vi "ActualizarFrecuencia.vi"(8 "error in (no error)":errorcluster, 11 "Prueba031 in":refnum<class "Prueba03.lvclass">) -> (0 "error out":errorcluster, 1 "newFrec":string, 3 "Prueba031 out":refnum<class "Prueba03.lvclass">)   [LabVIEW 2019, in "Prueba03.lvclass"]
uses:
  Prueba03.lvclass
  Prueba03.lvclass/Prueba03.ctl
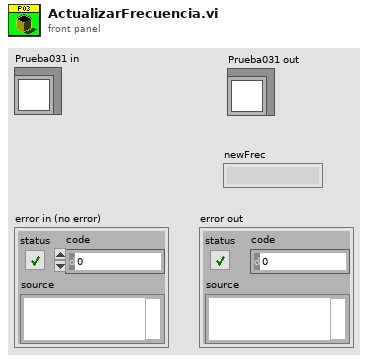
[diagram p1: front panel]
types:
  T1 = cluster{"ControlName":string, "ControlReference":refnum<vi>}[]
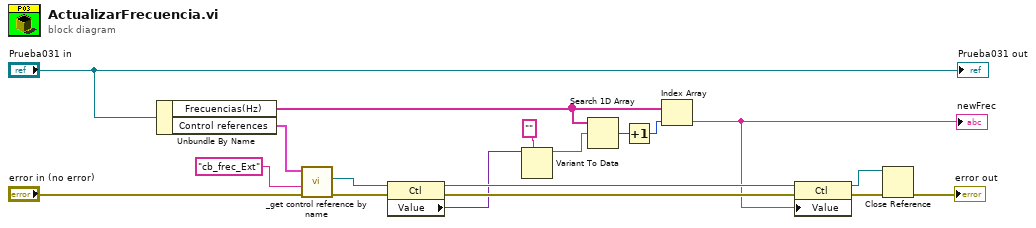
[diagram p0: block diagram]
diagram:
  n1 = Unbundle By Name("Prueba031 in") -> ("Frecuencias(Hz)"=w7:string[], "Control references"=w13:T1)
  n2 = call "_get control reference by name.vi"("error in (no error)"="error in (no error)", "Control name"="cb_frec_Ext", "Control references"=w13) -> ("error out"=w14:errorcluster, "Ctl Refnum"=w11:refnum<vi>)  [unwired: 3 in]
  n3 = property on="Property Node" class="Ctl"(reference=w11, error in=w14) -> (reference out=w10:refnum<vi>, error out=w16:errorcluster, "Value"=w9:variant)
  n4 = Variant To Data(type="" ("Control name"), Variant=w9) -> (data=w6:string)  [unwired: 1 in, 1 out]
  n5 = Search 1D Array(1D array=w7, element=w6) -> (index of element=w17:i32)  [unwired: 1 in]
  n6 = Increment(x=w17) -> (x+1=w18:i32)
  n7 = Index Array(array=w7, index=w18) -> (element=w4:string)
  "newFrec" <- w4
  n8 = property on="Property Node" class="Ctl"(reference=w10, error in=w16, "Value"=w4) -> (reference out=w3:refnum<vi>, error out=w2:errorcluster)
  n9 = Close Reference(reference=w3, error in (no error)=w2) -> (error out=→"error out":errorcluster)
  "Prueba031 out" <- "Prueba031 in"
